vi "Core.vi"(8 "error in (no error)":errorcluster, 10 "Path":path, 11 "ExcelReader in":refnum<class "ExcelReader.lvclass">) -> (0 "error out":errorcluster, 2 "MemberAttendance":refnum<class "MemberAttendance.lvclass">[](array[class]), 3 "ExcelReader out":refnum<class "ExcelReader.lvclass">)   [LabVIEW 2015, in "Admin_Actor.lvlib" / "ExcelReader.lvclass"]
uses:
  ExcelReader.lvclass
  MemberAttendance/MemberAttendance.lvclass
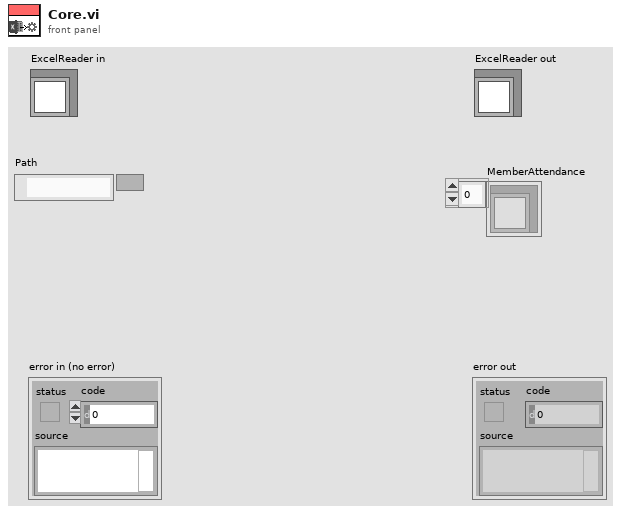
[diagram p1: front panel]
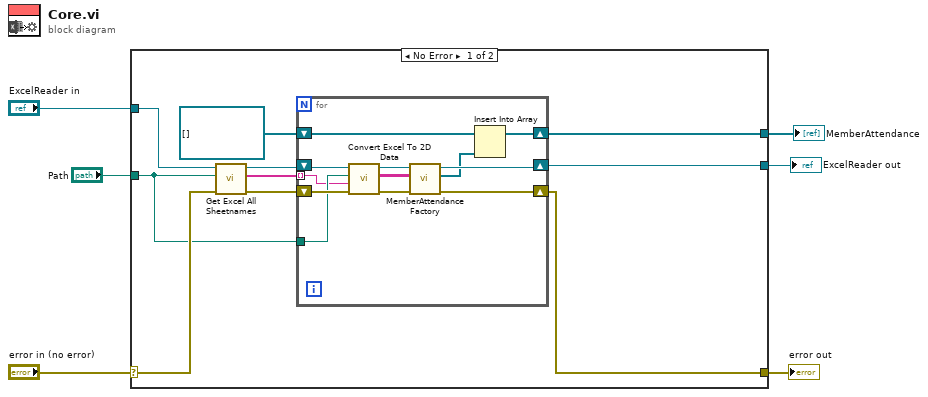
[diagram p0: block diagram]
diagram:
  n1 = case shown="No Error" "error in (no error)" {
    selector: "error in (no error)" -> [w15 w30]
    tunnel: [w10 w30] -> w5
    tunnel: [w9 w29] -> w3
    tunnel: "ExcelReader in" -> [w16 w29]
    tunnel: "Path" -> [w11 _]
    tunnel: [w7 _] -> w1
    frame No Error {
      n2 = call "Get Excel All Sheetnames.vi"("error in (no error)"=w15, "Path"=w11, "ExcelReader in"=w16) -> ("error out"=w12:errorcluster, "SheetNames(\"\")"=w14:string[], "ExcelReader out"=w13:refnum<class "ExcelReader.lvclass">)  [unwired: 6 in]
      n3 = for {
        tunnel: w14 -> [w17] mode=indexing
        tunnel: w11 -> [w26]
        shift-right: [w22] -> w9
        shift-left: w13 -> [w27]
        shift-right: [w21] -> w10
        shift-left: w12 -> [w28]
        shift-right: [w18] -> w7
        shift-left: refnum<class "MemberAttendance.lvclass">[] [] ("MemberAttendance") -> [w20]
        n4 = call "Convert Excel To 2D Data.vi"("error in (no error)"=w28, "SheetName(\"\")"=w17, "Path"=w26, "ExcelReader in"=w27) -> ("error out"=w24:errorcluster, "data"=w23:string[][], "ExcelReader out"=w25:refnum<class "ExcelReader.lvclass">)  [unwired: 5 in]
        n5 = call "MemberAttendance Factory.vi"("error in (no error)"=w24, "2D Data"=w23, "ExcelReader in"=w25) -> ("error out"=w21:errorcluster, "MemberAttendance"=w19:refnum<class "MemberAttendance.lvclass">[], "ExcelReader out"=w22:refnum<class "ExcelReader.lvclass">)  [unwired: 6 in]
        n6 = Insert Into Array(array=w20, new element=w19) -> (w18:refnum<class "MemberAttendance.lvclass">[])  [unwired: 1 in]
      }
    }
    frame Error {
    }
  }
  "error out" <- w5
  "ExcelReader out" <- w3
  "MemberAttendance" <- w1
